vi "data_add_array.vi"(9 "Data HEX string":string[](array[string]), 10 "Starting address char string":string, 11 "USB Interface Name":refnum<visa-resource-name>="COM3") -> ()   [LabVIEW 2012]
panel:
  out "Byte2":u8 format="%x"
  out "Byte1":u8 format="%x"
  out "Byte0":u8 format="%x"
  out "Starting Address Char":string
  out "Data Array Indicatro":string[](array[string])
  out "Address Array Indicator HEX":string[](array[string])
  # "HEX value of each byte"
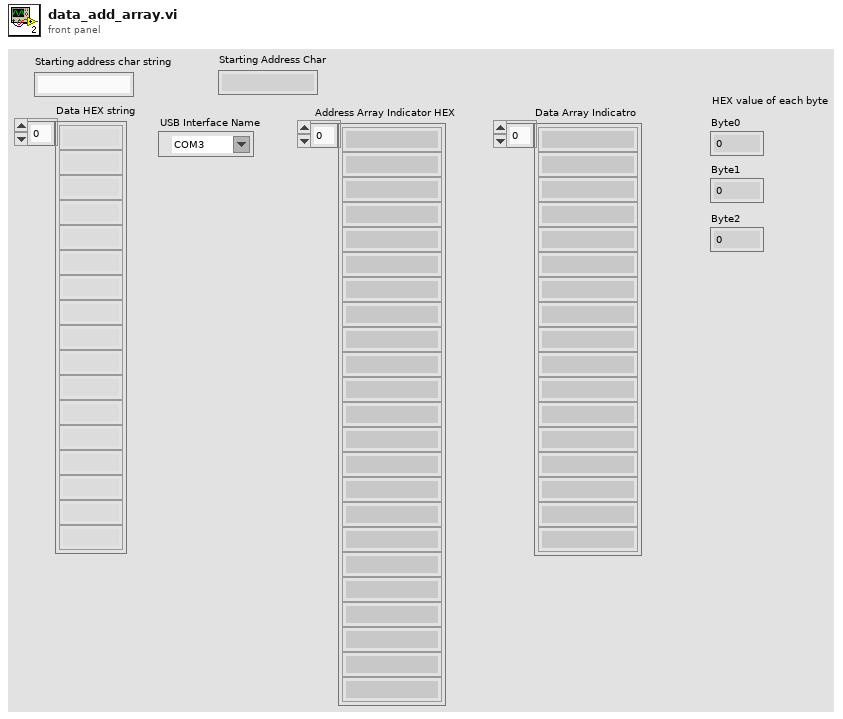
[diagram p1: front panel]
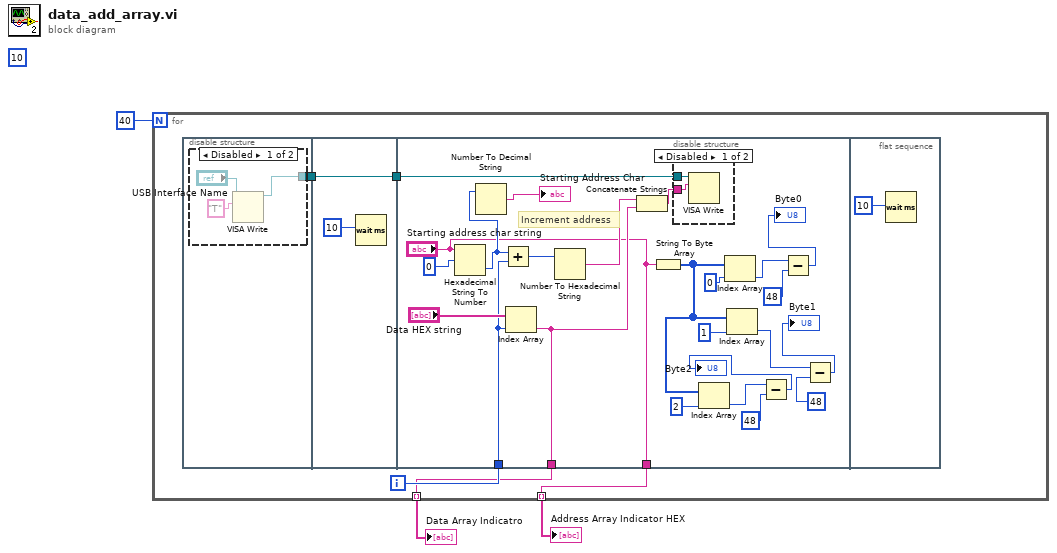
[diagram p0: block diagram]
diagram:
  (unwired) 10
  n1 = for {
    N: 40 -> [_]
    tunnel: [w7] -> w2 mode=indexing
    tunnel: [w6] -> w1 mode=indexing
    i -> [w8]
    n2 = flat-sequence {
      tunnel: [w9] -> w5
      tunnel: w5 -> [w14]
      tunnel: [w14] -> w4
      tunnel: w8 -> [w36]
      tunnel: ["Starting address char string"] -> w7
      tunnel: [w35] -> w6
      tunnel: w4 -> [w34]
      frame #0 {
        n3 = disable-structure shown="Disabled" {
          disable-tunnel: [w10 _] -> w9
          frame Disabled {
            n4 = VISA Write(VISA resource name="USB Interface Name", write buffer="T") -> (VISA resource name out=w10:refnum<visa-resource-name>)  [unwired: 1 in, 2 out]
          }
          frame Enabled {
          }
        }
      }
      frame #1 {
        n5 = Wait (ms)(milliseconds to wait=10) -> ()  [unwired: 1 out]
      }
      frame #2 {
        # "Increment address"
        n6 = Hexadecimal String To Number(string="Starting address char string", offset=0) -> (number=w30:u32)  [unwired: 1 in, 1 out]
        n7 = Number To Decimal String(number=w30) -> (decimal integer string=→"Starting Address Char":string)  [unwired: 1 in]
        n8 = Add(x=w30, y=w36) -> (x+y=w33:u32)
        n9 = Index Array(array="Data HEX string", index=w36) -> (element=w35:string)
        n10 = Number To Hexadecimal String(2:w33) -> (0:w25:string)  [unwired: 1 in]
        n11 = Concatenate Strings(w25, w35) -> (w37:string)
        n12 = String To Byte Array(string="Starting address char string") -> (unsigned byte array=w19:u8[])
        n13 = disable-structure shown="Disabled" {
          disable-tunnel: w37 -> [w39 _]
          disable-tunnel: w34 -> [w40 _]
          frame Disabled {
            n14 = VISA Write(VISA resource name=w40, write buffer=w39) -> ()  [unwired: 1 in, 3 out]
          }
          frame Enabled {
          }
        }
        n15 = Index Array(array=w19, index=2) -> (element=w17:u8)
        n16 = Index Array(array=w19, index=0) -> (element=w28:u8)
        n17 = Index Array(array=w19, index=1) -> (element=w21:u8)
        n18 = Subtract(x=w17, y=48) -> (x-y=→"Byte2":i32)
        n19 = Subtract(x=w28, y=48) -> (x-y=→"Byte0":i32)
        n20 = Subtract(x=w21, y=48) -> (x-y=→"Byte1":i32)
      }
      frame #3 {
        n21 = Wait (ms)(milliseconds to wait=10) -> ()  [unwired: 1 out]
      }
    }
  }
  "Address Array Indicator HEX" <- w2
  "Data Array Indicatro" <- w1
